vi "3-1 controllo se compreso IF AND (ex 2-1 control) difficile control.vi"(1 "control":bool, 2 "low limit":dbl(knob) scale=0.0..10.0 scale format="%.1f", 3 "hight limit":dbl(knob) scale=0.0..10.0 scale format="%.1f", 4 "data in":dbl format="%.2f") -> (0 "data out":dbl(knob) scale=0.0..10.0 scale format="%.1f")   [LabVIEW 2012]
panel:
  # "Se control = ON, bisogna verificare che il valore sia compreso nei limiti\n                     trasferendo il valore di ingresso diviso per il range ( hight limit-low limit)\n                     in uscita se ci˜ si verifica; in caso contrario o \nse control = OFF, non viene effettuato nessun controllo e il valore di ingresso passa\n                    direttamente in uscita"
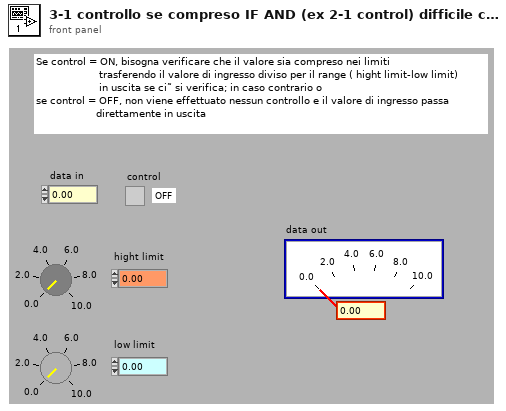
[diagram p1: front panel]
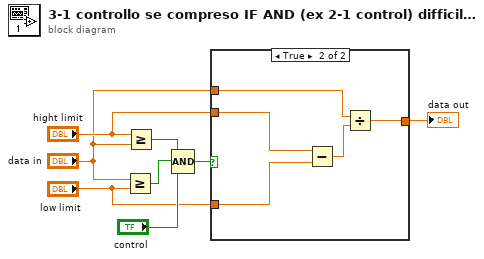
[diagram p0: block diagram]
diagram:
  n1 = Greater Or Equal?(x="data in", y="low limit") -> (x >= y?=w6:bool)
  n2 = Greater Or Equal?(x="hight limit", y="data in") -> (x >= y?=w7:bool)
  n3 = Compound Arithmetic op=AND(w7, w6, "control") -> (w4:bool)
  n4 = case shown="True" w4 {
    tunnel: "data in" -> [w9 w11]
    tunnel: [w9 w10] -> w8
    tunnel: "hight limit" -> [_ w13]
    tunnel: "low limit" -> [_ w12]
    frame False {
    }
    frame True {
      n5 = Subtract(x=w13, y=w12) -> (x-y=w14:dbl)
      n6 = Divide(x=w11, y=w14) -> (x/y=w10:dbl)
    }
  }
  "data out" <- w8
